vi "Arm.vi"(8 "error in (no error)":errorcluster, 9 "Request type":T1=enum."User command", 10 "Controller name":string, 11 "Pulse Driver in":refnum<class "Pulse Driver.lvclass">) -> (0 "error out":errorcluster, 3 "Pulse Driver out":refnum<class "Pulse Driver.lvclass">)   [LabVIEW 2021, in "Pulse Driver.lvclass"]
uses:
  Pulse Driver.lvclass
  Pulse Driver.lvclass/Pulse Driver.ctl
  LabActor/Controllers/Process Controller/Request type.ctl
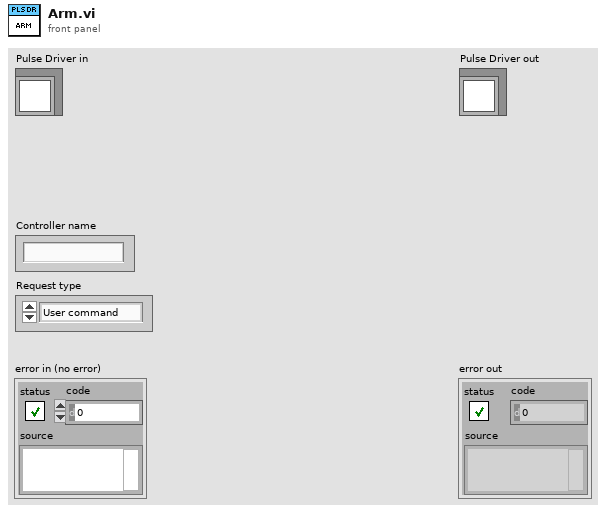
[diagram p1: front panel]
types:
  T1 = typedef "Request type.ctl" = enum16{"Process complete", "User command", "Auto-restart", "Error"}
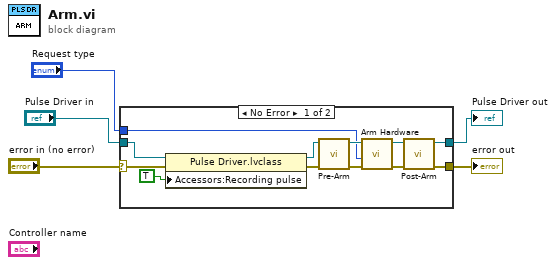
[diagram p0: block diagram]
diagram:
  n1 = case shown="No Error" "error in (no error)" {
    selector: "error in (no error)" -> [w10 w19]
    tunnel: [w8 w19] -> w4
    tunnel: [w7 w18] -> w2
    tunnel: "Pulse Driver in" -> [w9 w18]
    tunnel: "Request type" -> [w6 _]
    frame No Error {
      n2 = property class="Pulse Driver.lvclass"(reference=w9, error in=w10, "Accessors:Recording pulse"=TRUE ("Recording pulse")) -> (reference out=w12:refnum<class "Pulse Driver.lvclass">, error out=w11:errorcluster)
      n3 = call-dynamic "Pre-Arm.vi"("error in (no error)"=w11, "Pulse Driver in"=w12) -> ("error out"=w17:errorcluster, "Pulse Driver out"=w16:refnum<class "Pulse Driver.lvclass">)  [unwired: 8 in]
      n4 = call-dynamic "Arm Hardware.vi"("error in (no error)"=w17, "Request type"=w6, "Pulse Driver in"=w16) -> ("error out"=w15:errorcluster, "Pulse Driver out"=w14:refnum<class "Pulse Driver.lvclass">)  [unwired: 7 in]
      n5 = call-dynamic "Post-Arm.vi"("error in (no error)"=w15, "Pulse Driver in"=w14) -> ("error out"=w8:errorcluster, "Pulse Driver out"=w7:refnum<class "Pulse Driver.lvclass">)  [unwired: 8 in]
    }
    frame Error {
    }
  }
  "error out" <- w4
  "Pulse Driver out" <- w2
